vi "FT_Write_Byte_Data.vi"(8 "error in (no error)":errorcluster, 9 "Bytes To Write":u32, 10 "Buffer":u8[](array[numeric]), 11 "Handle":u64) -> (0 "error out":errorcluster, 1 "FT_Status":u32(ring) items=["FT_OK", "FT_INVALID_HANDLE", "FT_DEVICE_NOT_FOUND", "FT_DEVICE_NOT_OPENED", "FT_IO_ERROR", "FT_INSUFFICIENT_RESOURCES", "FT_INVALID_PARAMETER", "FT_INVALID_BAUD_RATE", "FT_DEVICE_NOT_OPENED_FOR_ERASE", "FT_DEVICE_NOT_OPENED_FOR_WRITE", "FT_FAILED_TO_WRITE_DEVICE", "FT_EEPROM_READ_FAILED", "FT_EEPROM_WRITE_FAILED", "FT_EEPROM_ERASE_FAILED", "FT_EEPROM_NOT_PRESENT", "FT_EEPROM_NOT_PROGRAMMED", "FT_INVALID_ARGS", "FT_NOT_SUPPORTED", "FT_OTHER_ERROR"], 2 "Bytes Written":u32, 3 "Handle Out":u64)   [LabVIEW 2018]
uses:
  FTD2XX.dll
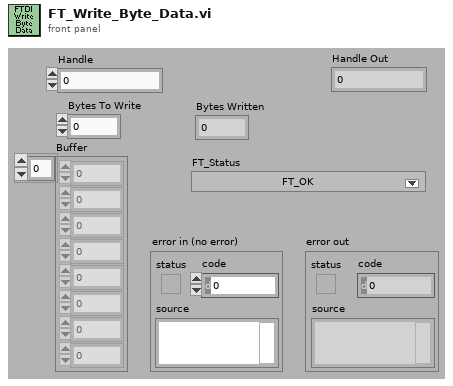
[diagram p1: front panel]
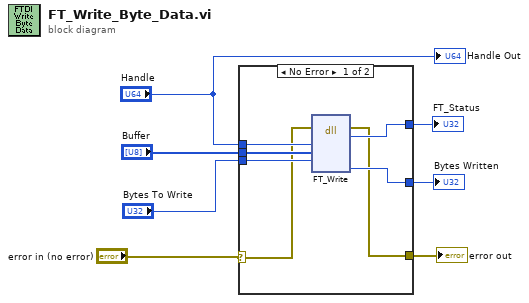
[diagram p0: block diagram]
diagram:
  n1 = case shown="No Error" "error in (no error)" {
    selector: "error in (no error)" -> [w9 w15]
    tunnel: [w14 _] -> w7
    tunnel: "Handle" -> [w13 _]
    tunnel: "Bytes To Write" -> [w12 _]
    tunnel: [w11 _] -> w5
    tunnel: "Buffer" -> [w10 _]
    tunnel: [w8 w15] -> w2
    frame No Error {
      n2 = dll-call lib="FTD2XX.dll" fn="FT_Write"(error in=w9, "Handle"=w13, "Buffer"=w10, "BytesToWrite"=w12) -> (error out=w8:errorcluster, "FT_Status"=w14:u32, "BytesWritten"=w11:u32)  [unwired: 6 in, 1 out]
    }
    frame Error {
    }
  }
  "FT_Status" <- w7
  "Bytes Written" <- w5
  "error out" <- w2
  "Handle Out" <- "Handle"
